vi "DAQ.Read AI.vi"(8 "error in":errorcluster, 11 "Instrument.DAQ in":refnum<class "Instrument.DAQ.lvclass">) -> (0 "error out":errorcluster, 2 "AI []":waveform(dbl)[](array[waveform]), 3 "Instrument.DAQ out":refnum<class "Instrument.DAQ.lvclass">, 4 "AI time (s)":dbl=2.0)   [LabVIEW 2019, in "Instrument.Lockin.lvlib" / "Instrument.DAQ.lvclass"]
uses:
  Instrument.DAQ.lvclass
  Instrument.DAQ.lvclass/Instrument.DAQ.ctl
  Typedefs/Simulation Mode--enum.ctl
  Simulate/Waveguide Model--Cluster.ctl
  Generator/Generator.lvclass
panel:
  in  "show graph?":bool
  out "Waveform Graph":waveform(dbl)[](graph)
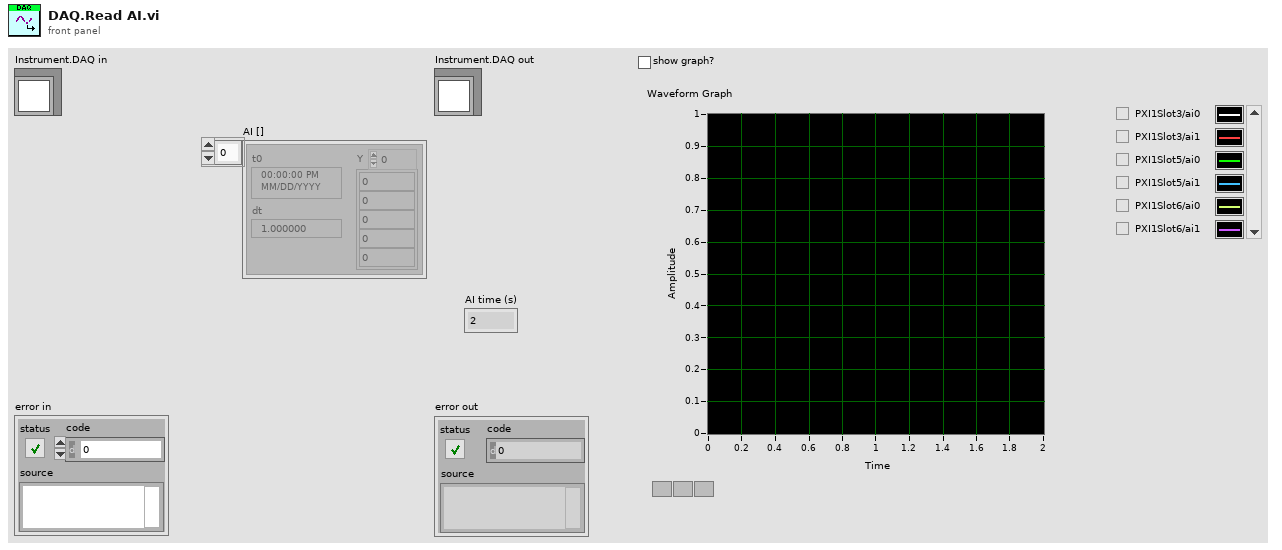
[diagram p1: front panel]
types:
  T1 = typedef "Instrument.Lockin.lvlib/Instrument.DAQ.lvclass/Simulation Mode--enum.ctl" = enum16{"AI = HW simulated", "AI = noise*AO", "AI = waveguide"}
  T2 = typedef "Instrument.Lockin.lvlib/Instrument.DAQ.lvclass/DeviceInfo--Cluster.ctl" = cluster{"DeviceName":string, "DevIsSimulated":bool, "DeviceSerialNumber":string, "ProductType":string, "ProductCategory":i32, "ProductNumber":u32, "ChassisNumber":u32, "SlotNumber":u32, "ChassisName":string, "ChassisSerialNumber":string, "DevTemp":dbl, "SelfCal.LastDate/Time":string, "SelfCal.LastTemp":dbl, "calibration due?":bool}
  T3 = typedef "Instrument.Lockin.lvlib/Instrument.DAQ.lvclass/Waveguide Model--Cluster.ctl" = cluster{"I+":i32, "I-":i32, "V+":i32, "V-":i32, "Vsg":i32}
  T4 = typedef "Instrument.Lockin.lvlib/Instrument.DAQ.lvclass/AI.Channel--Cluster--Array.ctl" = T5[]
  T5 = typedef "Instrument.Lockin.lvlib/Instrument.DAQ.lvclass/AI.Channel--Cluster.ctl" = cluster{"Enable?":bool, "Channel":i32, "References":u16[], "reference index":i32}
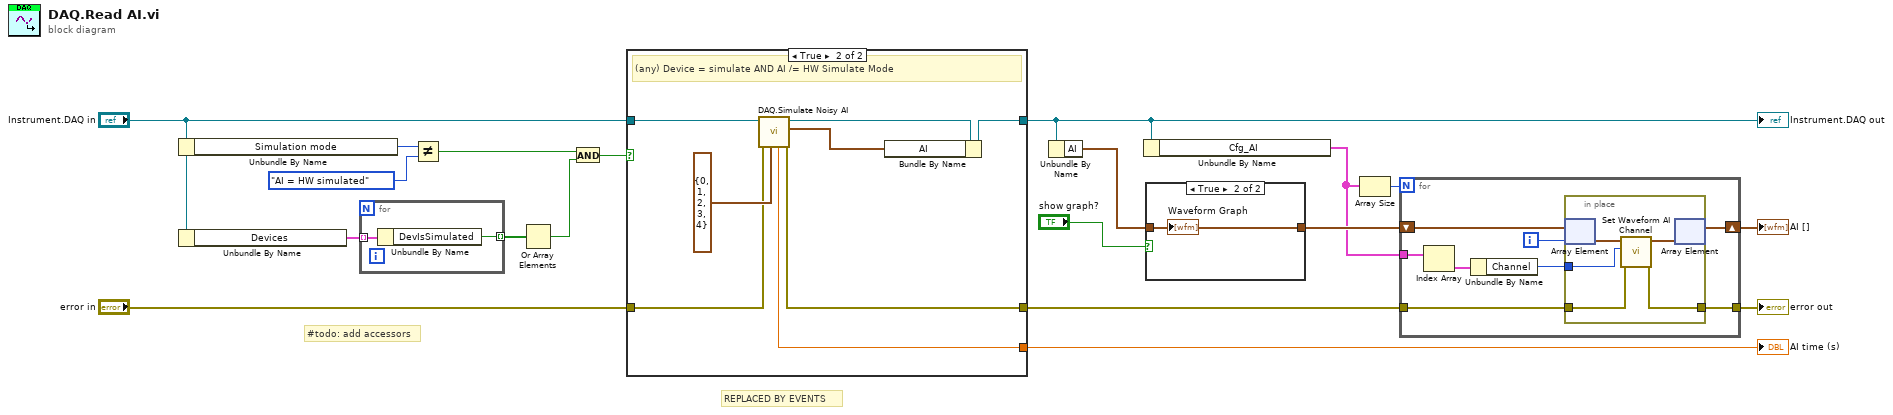
[diagram p0: block diagram]
diagram:
  # "REPLACED BY EVENTS"
  # "#todo: add accessors"
  n1 = Unbundle By Name("Instrument.DAQ in") -> ("Simulation mode"=w13:T1)
  n2 = Unbundle By Name("Instrument.DAQ in") -> ("Devices"=w6:T2[])
  n3 = for {
    tunnel: w6 -> [w21] mode=indexing
    tunnel: [w20] -> w5 mode=indexing
    n4 = Unbundle By Name(w21) -> ("DevIsSimulated"=w20:bool)
  }
  n5 = Not Equal?(x=w13, y=Simulation_Mode--enum."AI = HW simulated") -> (x != y?=w2:bool)
  n6 = Or Array Elements(Boolean array=w5) -> (logical OR=w4:bool)
  n7 = And(x=w2, y=w4) -> (x .and. y?=w3:bool)
  n8 = case shown="True" w3 {
    tunnel: "error in" -> [w22 w29]
    tunnel: [w22 w28] -> w12
    tunnel: "Instrument.DAQ in" -> [w23 w31]
    tunnel: [w23 w25] -> w8
    tunnel: [_ w24] -> w11
    frame False {
      # "Device /= simulate OR AI = HW simulated mode"
    }
    frame True {
      # "(any) Device = simulate AND AI /= HW Simulate Mode"
      n9 = call "DAQ.Simulate Noisy AI.vi"("Waveguide Cluster"=T3 {"I+"=0, "I-"=1, "V+"=2, "V-"=3, "Vsg"=4}, "error in (no error)"=w29, "Instrument.DAQ in"=w31) -> ("error out"=w28:errorcluster, "Noisy Signal Graph"=w27:waveform(dbl)[], "Instrument.DAQ out"=w26:refnum<class "Instrument.DAQ.lvclass">, "AI time (s)"=w24:dbl)  [unwired: 5 in]
      n10 = Bundle By Name(cluster=w26, "AI"=w27) -> (w25:refnum<class "Instrument.DAQ.lvclass">)
    }
  }
  "Instrument.DAQ out" <- w8
  "AI time (s)" <- w11
  n11 = Unbundle By Name(w8) -> ("AI"=w19:waveform(dbl)[])
  n12 = Unbundle By Name(w8) -> ("Cfg_AI"=w15:T4)
  n13 = case shown="True" "show graph?" {
    tunnel: w19 -> [w32 w33]
    tunnel: [w32 w33] -> w18
    frame False {
    }
    frame True {
      "Waveform Graph" <- w33
    }
  }
  n14 = Array Size(array=w15) -> (size(s)=w14:i32)
  n15 = for {
    N: w14 -> [_]
    tunnel: w15 -> [w34]
    tunnel: w12 -> [w39]
    tunnel: [w38] -> w17
    shift-right: [w37] -> w16
    shift-left: w18 -> [w40]
    i -> [w41]
    n16 = Index Array(array=w34) -> (element=w35:T5)  [unwired: 1 in]
    n17 = Unbundle By Name(w35) -> ("Channel"=w36:i32)
    n18 = in-place {
      in-place-border: w39 -> [w44]
      in-place-border: [w43] -> w38
      in-place-border: w36 -> [w42]
      n19 = in-place-array #1(w40, w41) -> (w46:waveform(dbl))
      n20 = call "Set Waveform AI Channel.vi"("error in (no error)"=w44, "AI Channel"=w42, "Waveform in"=w46) -> ("error out"=w43:errorcluster, "Waveform out"=w45:waveform(dbl))  [unwired: 7 in]
      n21 = in-place-array #1(w45) -> (w37:waveform(dbl)[])  [unwired: 1 out]
    }
  }
  "error out" <- w17
  "AI []" <- w16
